vi "_22_Sample_qsns_10[2].vi"() -> ()   [LabVIEW 2020]
panel:
  out "Array":i32[](array[numeric])
  out "x-y":i32
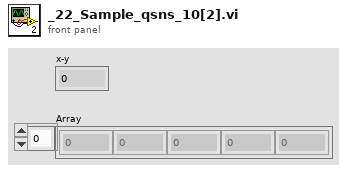
[diagram p1: front panel]
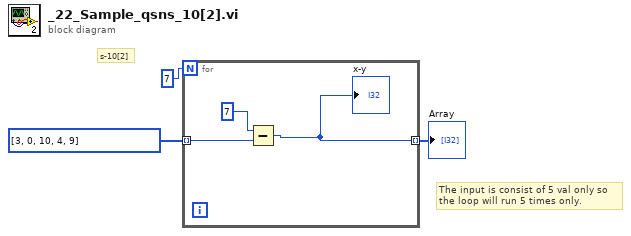
[diagram p0: block diagram]
diagram:
  # "The input is consist of 5 val only so \nthe loop will run 5 times only."
  # "s-10[2]"
  n1 = for {
    N: 7 -> [_]
    tunnel: i32[] [3, 0, 10, 4, 9] -> [w6] mode=indexing
    tunnel: [w4] -> w1 mode=indexing
    n2 = Subtract(x=7, y=w6) -> (x-y=w4:i32)
    "x-y" <- w4
  }
  "Array" <- w1
